vi "LV to ITX XY AutoPlot.vi"(0 "filename":string="datatest", 1 "path":path=path "C:/Users/voodoo.SEAGATE/Desktop/datatest", 5 "Notes":string, 7 "XY Array":cluster{"X  array":dbl[], "Y  Array":dbl[]}[](array[cluster])=[{"X  array"=[0.5, 0.4998, 0.4999, 0.4999, 0.5236, 0.4256, 0.4962, 0.4959, 0.4966, 0.494, 0.4885, 0.4829, 0.4742, 0.4661, 0.457, 0.4476, 0.4352, 0.4231, 0.4109, 0.3956, 0.3784, 0.3627, 0.3484, 0.3292, 0.3131, 0.294, 0.2787, 0.262, 0.2463, 0.2317, 0.2178, 0.2049, 0.1939, 0.187, 0.1807, 0.1769, 0.1717, 0.168, 0.1643, 0.1612, 0.158, 0.1553, 0.1526, 0.1504, 0.1481, 0.1459, 0.144, 0.142, 0.1408, 0.139, 0.1371, 0.1359, 0.1345, 0.133, 0.1318, 0.1304, 0.1293, 0.1284, 0.1269, 0.1259, 0.125, 0.1239, 0.1228, 0.1218, 0.1208, 0.1199, 0.1191, 0.1183, 0.1174, 0.1167, 0.1159, 0.115, 0.1144, 0.1137, 0.113, 0.1122, 0.1113, 0.1106, 0.1097, 0.109, 0.1082, 0.1076, 0.1068, 0.106, 0.1054, 0.1046, 0.104, 0.1034, 0.1029, 0.1022, 0.1016, 0.101, 0.1006, 0.099889, 0.099452, 0.098819, 0.098203, 0.097827, 0.097362, 0.096717, 0.096282, 0.095797, 0.095203, 0.094792, 0.094216, 0.09387, 0.093405, 0.092786, 0.092322, 0.091812, 0.091285, 0.090909, 0.090377, 0.08989, 0.089323, 0.088888, 0.088471, 0.08797, 0.087655, 0.087169, 0.086802, 0.086242, 0.085927, 0.085399, 0.084991, 0.084619, 0.084185, 0.083826, 0.083393, 0.083078, 0.082648, 0.082294, 0.081803, 0.081596, 0.081148, 0.080761, 0.080401, 0.079989, 0.079653, 0.079248, 0.078921, 0.078589, 0.07814, 0.077823, 0.077558, 0.077106, 0.076804, 0.076394, 0.076062, 0.075777, 0.075425, 0.07514, 0.074776, 0.074486, 0.074122, 0.073813, 0.073502, 0.073138, 0.072894, 0.072625, 0.072343, 0.071954, 0.071672, 0.071319, 0.071071, 0.070745, 0.070523, 0.070176, 0.069888, 0.069549, 0.069194, 0.069007, 0.068719, 0.068417, 0.068136, 0.06789, 0.067624, 0.067354, 0.067084, 0.066854, 0.066573, 0.066332, 0.066031, 0.06589, 0.06564, 0.065397, 0.065044, 0.064902, 0.06465, 0.064367, 0.064115, 0.063955, 0.063744, 0.063583, 0.063306, 0.063125, 0.062917, 0.062634, 0.062453, 0.062225, 0.061985, 0.061769, 0.06153, 0.061364, 0.061192, 0.06103, 0.060759, 0.060543, 0.060413, 0.060208, 0.060005, 0.059814, 0.059682, 0.059481, 0.059335, 0.059177, 0.058964, 0.058819, 0.058697, 0.058529, 0.058358, 0.05824, 0.058121, 0.057938, 0.05779, 0.057655, 0.057469, 0.057371, 0.057247, 0.05707, 0.056951, 0.056731, 0.056673, 0.056531, 0.056397, 0.056241, 0.056174, 0.055959, 0.05586, 0.055687, 0.055558, 0.055436, 0.055357, 0.055172, 0.055022, 0.054945, 0.054822, 0.054671, 0.054565, 0.054397, 0.054258, 0.054166, 0.054032, 0.05393, 0.053787, 0.053728, 0.053536, 0.053427, 0.053317, 0.053231, 0.053077, 0.052944, 0.052818, 0.0527, 0.052558, 0.052416, 0.052299, 0.052192, 0.052072, 0.051964, 0.051846, 0.051768, 0.051588, 0.051465, 0.051397, 0.051221, 0.051115, 0.051005, 0.050915, 0.050775, 0.050667, 0.050538, 0.050424, 0.050301, 0.050197, 0.050106, 0.050014, 0.049935, 0.049786, 0.049702, 0.049626, 0.049529, 0.049441, 0.049454, 0.049514, 0.049568], "Y  Array"=[23165.718345688696, 23653.128800246926, 23300.55102100627, 23740.83856952551, 24076.906035910855, 23468.196302062795, 21799.2522815103, 22057.998271040688, 22074.593013844787, 22636.877593082056, 23615.114150003326, 23028.446549699478, 22873.118627884818, 23608.236549277237, 23200.501086717766, 23931.64887307282, 22903.559950206767, 24385.00434402636, 23815.977936449555, 23262.90176433917, 22746.029144306794, 22812.13176732137, 22698.822083516177, 22590.365126675086, 23372.57915720584, 21421.873047831912, 21420.252100832775, 22107.695491672286, 21431.064022092916, 21531.12664561267, 20850.211606366014, 21597.605339082318, 19403.464393329552, 19842.902488342836, 21272.243333499086, 20437.763820512533, 19089.059824795968, 19400.513216843112, 17993.476827448274, 17947.768926517805, 16845.2229378802, 16934.941541792552, 15221.45141515402, 14840.21339782445, 15731.770162488005, 14730.470316007568, 13268.927651243152, 13182.884929505231, 12828.65977258054, 12108.027135394115, 12690.166315209592, 11366.45314734667, 12558.223438809795, 11591.955522281545, 12169.596854776473, 10149.071383974924, 11201.298769784791, 11737.53551661967, 10356.919262495834, 10966.576569298053, 10906.208691869273, 10105.524500963105, 11036.881512404618, 11433.694756583182, 11026.773755834432, 9899.84830214666, 10354.86909547578, 10551.846026866433, 10412.971643033581, 10174.034733242972, 9349.626337088881, 10308.38322838087, 9262.049689681395, 10011.710366956248, 9216.19750315671, 9184.867364310348, 9820.355427150502, 10161.734926471918, 9877.979844582393, 9015.633364252575, 10604.333372193434, 10205.273816290917, 9309.00792800317, 9520.423096393997, 9033.272437712472, 9212.181979709794, 9789.887074618226, 10040.61435526264, 9676.454811321963, 8555.390251065968, 9464.78146147957, 9098.752970985668, 9072.558969049674, 9606.312070074478, 9056.427348975485, 8750.9555518609, 10032.070191590072, 8911.368790158516, 8524.557875241282, 9059.243502032157, 9584.686860730037, 9228.882243831715, 9741.423929410583, 9417.560871203685, 9304.421440357164, 9441.00963195965, 9696.541526722493, 9751.545542190133, 8676.94872084638, 8856.216515949756, 9208.99237956053, 9044.514996659176, 9313.961553374993, 8720.628628892886, 8995.477896818982, 9718.905136687794, 8790.024875837933, 8290.50475897958, 9346.333336469557, 9297.10703229354, 9194.650451226546, 9607.844623776677, 8488.429269134203, 9088.972278765983, 8830.703382924978, 9605.91677858658, 9216.032215244524, 9981.431207407706, 8697.77441310007, 8274.979314592363, 8420.33867794508, 8472.425850051453, 8525.535854313142, 9360.966352797253, 8966.745026142818, 8442.16543638555, 8329.574013042824, 7780.126632301061, 8438.803597540877, 8291.911663950963, 8582.061432875127, 8973.551656259286, 9321.056196048174, 8153.349784716115, 9049.48799862552, 8708.12130185736, 8546.633923505877, 8499.679002001654, 8740.002445439311, 8391.015012884383, 9219.095963274223, 7777.701643799162, 8312.977867851761, 9223.753001530184, 8993.798819644555, 8983.355799817195, 8009.789010490335, 8487.52832825222, 9040.181067471432, 9262.903050582656, 7885.087899787207, 8755.159511532851, 8196.24727759012, 9150.526456862883, 9817.869278781725, 8137.5034787333525, 8511.36699705151, 8657.20202264442, 7380.497375498042, 7784.48058223125, 8825.241623538739, 7754.396056839032, 8688.096703565447, 9362.783860247595, 8781.884411838177, 7843.704925708325, 8059.5077602254005, 8606.352198788965, 7776.027823433382, 8762.73986338239, 8725.951121681417, 8320.47723999792, 8710.685197192626, 8208.14396235819, 8101.347280692269, 8652.500637873336, 7988.528799407512, 9270.902406308685, 7963.051146685747, 8400.935021006599, 8608.050083557177, 8902.211224302813, 8372.445162067768, 7977.362281819596, 7613.905826867788, 7912.759710144272, 8599.861765881935, 8179.268257168343, 8601.817038918723, 8605.137929026116, 8636.388041149547, 8411.525691006766, 8871.903800808725, 7781.123300591914, 9058.337756810253, 8240.902893239163, 8784.228788972772, 8571.61697526162, 8119.420853773818, 8104.249660655999, 8803.788297140602, 8884.239972165173, 9015.72641481132, 8304.431415512656, 8658.449101132997, 9110.584432271182, 8406.832346477351, 8130.075504467065, 8185.687040062772, 9358.9726832901, 9088.1562053183, 8237.428414509348, 8929.48922228839, 8061.815654756303, 8254.57332017452, 8211.857674811881, 8059.284814631164, 8005.202474430426, 7819.959949932711, 8021.775067386229, 8294.298806005965, 7432.519832797439, 8225.048327287943, 7833.19653770287, 8680.325285616696, 8702.969138895349, 9004.018661116583, 7977.988709469854, 7939.282233243148, 8334.28655215735, 9229.14109996092, 8867.613897978074, 8401.449523945277, 7399.201371921939, 8033.1090112222155, 8859.703933764944, 8676.92519047193, 7975.820081704094, 7779.397269977999, 8171.658652375199, 7727.943052615354, 7588.814218487658, 8215.780094572254, 8610.477401317867, 8103.678311552077, 8825.270293415102, 7786.278736109644, 7834.627297664257, 8385.6397942722, 8173.396087918111, 8057.18085884151, 8551.588205771792, 8294.513419537629, 8747.659382990716, 8158.118782154173, 7727.493768867023, 7592.696442933768, 8859.192033733323, 7773.808337023467, 7738.1820326035595, 8015.454548215039, 8302.292810326826, 8466.787641571531, 8412.151028999333, 8422.044485856939, 7581.439140697347, 8196.542604030386, 8733.279719103077, 8807.032550899325, 8044.54473540655, 7709.161191961498, 8622.419182205638, 8002.8832648356765, 7546.354695629521, 8538.435040541328, 8316.077600700659, 7902.218737115643, 8427.056561648156, 7976.323284393145, 8011.003433368622, 8796.834976169688, 8049.140830931177, 8767.087781641521, 8670.408555294609, 8346.845105255541, 7928.9072543974]}], 11 "wavenames (.Vx, etc)":string[](array[string])=["Plot 0"], 12 "X,Y Labels":string[](array[string])=["x label", "y label"], 13 "X,Y Log":i32[](array[numeric])) -> (4 "file":path=path "C:/Users/voodoo.SEAGATE/Desktop/datatest/datatest.000019.itx")   [LabVIEW 2011]
doc: "Write your XY data to ITX file. This AutoPlot VI adds commands to automatically create a graph in Igor to quickly view your data.\n\n-- path: base path to save data\n-- filename: base filename\n-- Notes: add any notes here to help you remember what experiment you did\n-- XY Array: Array of Clusters (ie, Array of XY graphs)\n-- wavenames: Give each data array a unique name such as \"time, bias, current,...\"\n-- X,Y Labels: For plotting in Igor. Can be ignored.\n-- X,Y Log: Do you wan to show X or Y on Log scale in Igor?"
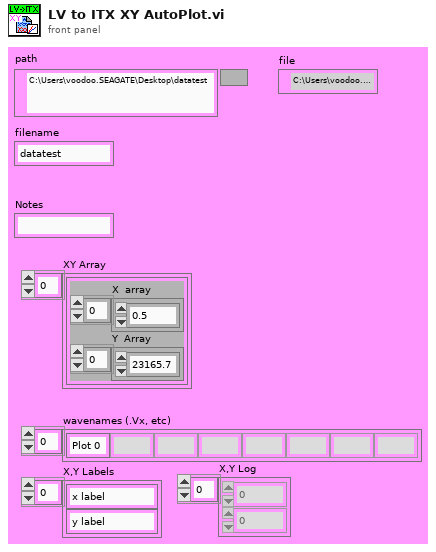
[diagram p1: front panel]
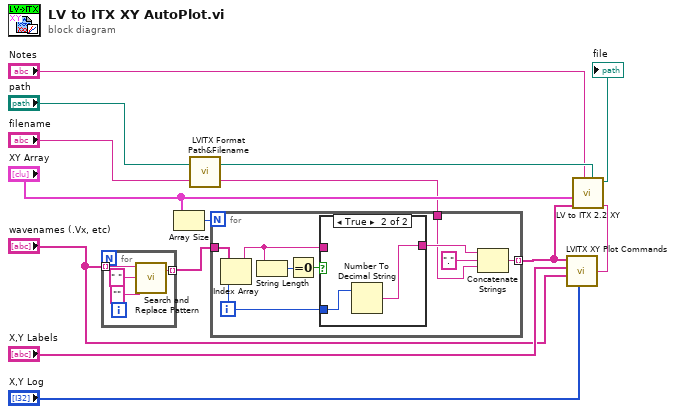
[diagram p0: block diagram]
diagram:
  n1 = for {
    tunnel: "wavenames (.Vx, etc)" -> [w16] mode=indexing
    tunnel: [w15] -> w4 mode=indexing
    n2 = call <vilib>:"Search and Replace Pattern.vi"("string"=w16, "regular expression (\"\")"=" " ("regular expression (\"\")"), "replace string (\"\")"="" ("replace string (\"\")")) -> ("result string"=w15:string)  [unwired: 2 in, 1 out]
  }
  n3 = Array Size(array="XY Array") -> (size(s)=w3:i32)
  n4 = call "LVITX Format Path&Filename.vi"("filename"="filename", "path"="path") -> ("file name without extension"=w2:string, "dup file"=w10:path)
  n5 = for {
    N: w3 -> [_]
    tunnel: w4 -> [w22]
    tunnel: w2 -> [w19]
    tunnel: [w27] -> w1 mode=indexing
    i -> [w23]
    n6 = Index Array(array=w22, index=w23) -> (element=w21:string)
    n7 = String Length(string=w21) -> (length=w24:i32)
    n8 = Equal To 0?(x=w24) -> (x = 0?=w25:bool)
    n9 = case shown="True" w25 {
      tunnel: w23 -> [_ w29]
      tunnel: [w28 w30] -> w20
      tunnel: w21 -> [w28 _]
      frame False {
      }
      frame True {
        n10 = Number To Decimal String(number=w29) -> (decimal integer string=w30:string)  [unwired: 1 out]
      }
    }
    n11 = Concatenate Strings(w20, "." ("string"), w19) -> (w27:string)
  }
  n12 = call "LVITX XY Plot Commands.vi"("X,Y Log"="X,Y Log", "Plot labels"="wavenames (.Vx, etc)", "X,Y Labels"="X,Y Labels", "wavenames"=w1) -> ("result string"=w12:string)  [unwired: 2 in]
  n13 = call "LV to ITX 2.2 XY.vi"("Commands"=w12, "filename"=w10, "Notes"="Notes", "wavenames"=w1, "XY Array"="XY Array") -> ("file"=→"file":path)  [unwired: 6 in]
